vi "log_subVI.vi"(2 "Ampiezza Min":string, 3 "freq ad ampiezza max":string, 4 "freq ad ampiezza min":string, 5 "Boolean 2":bool, 6 "Ampiezza Max":string, 7 "time stamp":timestamp) -> (0 "Formatted String Output":string[](array[string]))   [LabVIEW 2018]
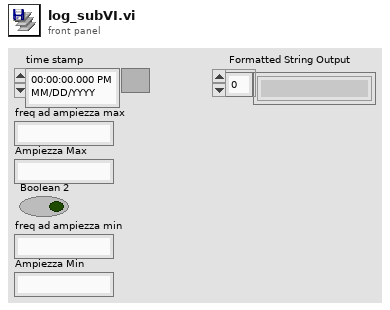
[diagram p1: front panel]
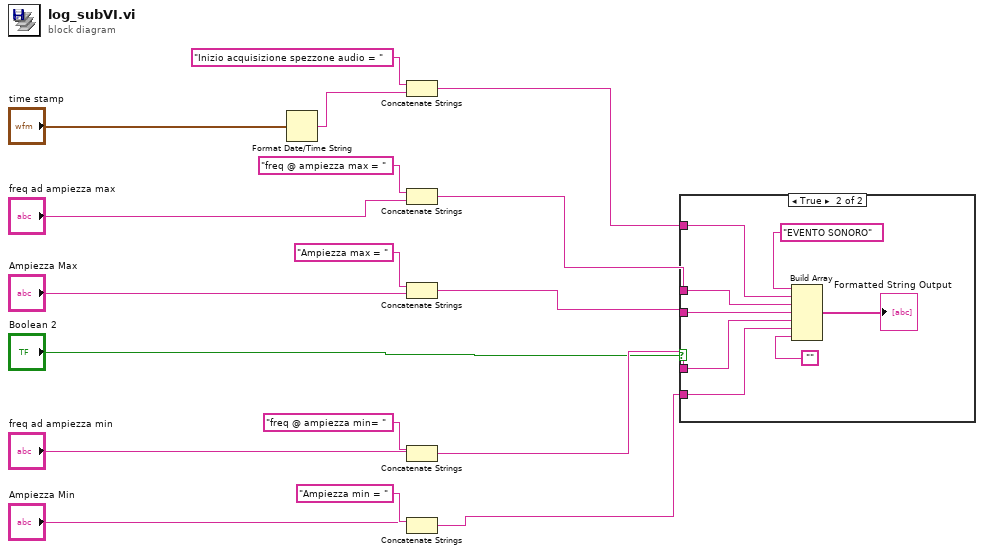
[diagram p0: block diagram]
diagram:
  n1 = Format Date/Time String(seconds (now)="time stamp") -> (date/time string=w12:string)  [unwired: 2 in]
  n2 = Concatenate Strings("Inizio acquisizione spezzone audio = " ("string"), w12) -> (w10:string)
  n3 = Concatenate Strings("freq @ ampiezza max = " ("string"), "freq ad ampiezza max") -> (w9:string)
  n4 = Concatenate Strings("Ampiezza max = " ("string"), "Ampiezza Max") -> (w8:string)
  n5 = Concatenate Strings("freq @ ampiezza min= " ("string"), "freq ad ampiezza min") -> (w7:string)
  n6 = Concatenate Strings("Ampiezza min = " ("string"), "Ampiezza Min") -> (w6:string)
  n7 = case shown="True" "Boolean 2" {
    tunnel: w10 -> [_ w25]
    tunnel: w9 -> [_ w24]
    tunnel: w8 -> [_ w23]
    tunnel: w7 -> [_ w22]
    tunnel: w6 -> [_ w21]
    frame False {
    }
    frame True {
      n8 = Build Array("EVENTO SONORO" ("string"), w25, w24, w23, w22, w21, "") -> (→"Formatted String Output":string[])
    }
  }
